vi "Actor UI.vi"   [LabVIEW 2020]
uses:
  <vilib>/ActorFramework/Stop Msg/Stop Msg.lvclass
  <vilib>/ActorFramework/Actor/Actor.lvclass
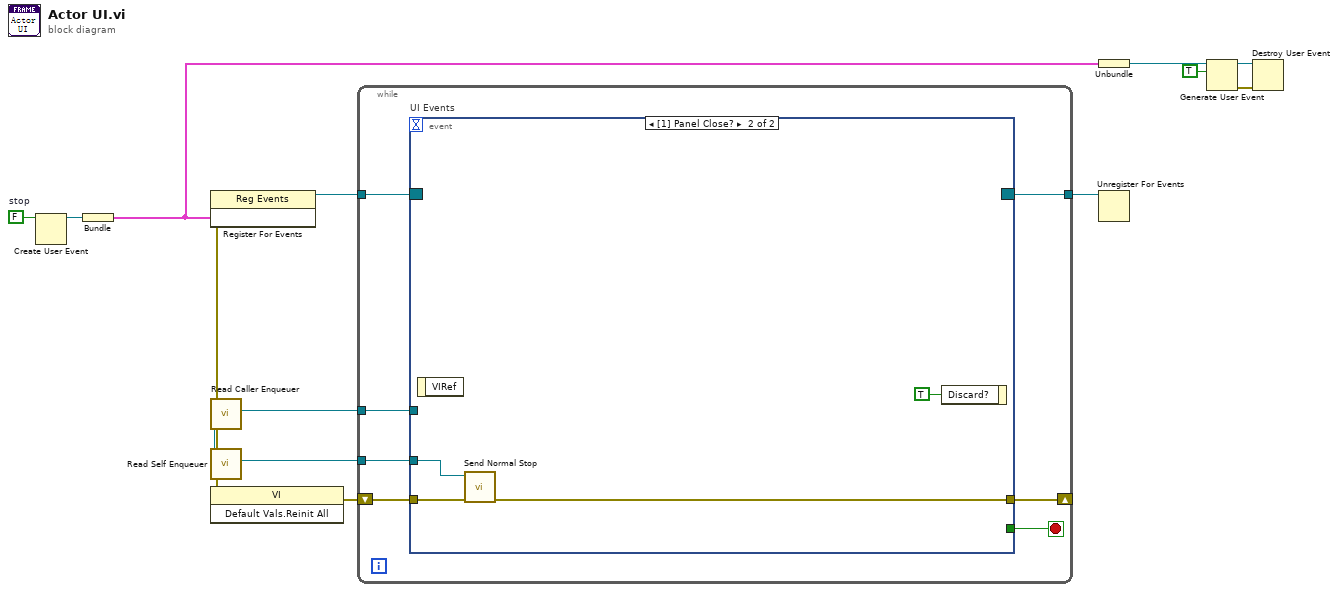
[diagram p0: block diagram]
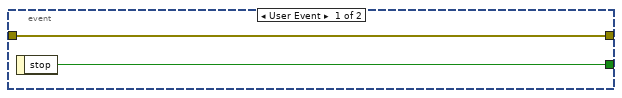
[diagram p2: hidden frame]
diagram:
  w10 = FALSE  # stop
  n1 = Create User Event(user event datatype=w10) -> (user event=w7:refnum<user-event>)  [unwired: 1 in, 1 out]
  n2 = Bundle("stop"=w7) -> (w6:cluster{"stop":refnum<user-event>})  [unwired: 1 in]
  n3 = register-events ("Main Register for Events")(w6) -> (reference out=w15:refnum<event-registration>, error in=w2:errorcluster)  [unwired: 1 in, 1 out]
  n4 = call <vilib>:"Read Self Enqueuer.vi"() -> ("Self Enqueuer"=w13:refnum<class "Message Enqueuer.lvclass">, "Actor"=w1:refnum<class "Actor.lvclass">)  [unwired: 10 in]
  n5 = call <vilib>:"Read Caller Enqueuer.vi"("Actor"=w1) -> ("Caller Enqueuer"=w12:refnum<class "Message Enqueuer.lvclass">)  [unwired: 10 in]
  n6 = invoke class="VI" method="Default Vals.Reinit All"(error in=w2) -> (error out=w11:errorcluster)  [unwired: 2 in, 2 out]
  n7 = while {
    tunnel: w15 -> [w22]
    tunnel: [w20] -> w14
    tunnel: w13 -> [w19]
    tunnel: w12 -> [w16]
    shift-right: [w17] -> _
    shift-left: w11 -> [w18]
    stop <- w21 stop-if-true
    n8 = event "UI Events" shown="[1] Panel Close?" {
      selector: w22 -> [_ _]
      dyn-events: [_ _] -> w20
      timeout: _ -> [_ _]
      tunnel: [w23 _] -> w21
      tunnel: w19 -> [_ w27]
      tunnel: w18 -> [w24 w26]
      tunnel: [w24 w25] -> w17
      tunnel: w16 -> [_ _]
      event User Event {
        n9 = event-data() -> ("stop"=w23:bool)  [unwired: 1 in]
      }
      event Panel Close? {
        n10 = event-data() -> ()  [unwired: 1 in, 1 out]
        n11 = call <vilib>:"Send Normal Stop.vi"("error in (no error)"=w26, "Message Enqueuer"=w27) -> ("error out"=w25:errorcluster)  [unwired: 9 in]
        n12 = event-data("Discard?"=TRUE) -> ()  [unwired: 1 in, 1 out]
      }
    }
  }
  n13 = Unbundle(w6) -> ("stop"=w5:refnum<user-event>)
  n14 = Unregister For Events(event registration refnum=w14) -> ()  [unwired: 1 in, 1 out]
  n15 = Generate User Event(user event=w5, event data cluster=TRUE ("event data")) -> (error in=w3:errorcluster, user event out=w8:refnum<user-event>, error out=w4:errorcluster)  [unwired: 1 in]
  n16 = Destroy User Event(user event=w8, error in=w4) -> ()  [unwired: 1 out]
